vi "Read Gain Values.vi"(6 "error in":errorcluster, 8 "MaxRead":i32, 9 "Channel in":u16) -> (0 "error out":errorcluster, 1 "Messages":T2(array[cluster]) {"ID" format="%.0x"; "DATA[0]" format="%.0x"; "DATA[1]" format="%.0x"; "DATA[2]" format="%.0x"; "DATA[3]" format="%.0x"; "DATA[4]" format="%.0x"; "DATA[5]" format="%.0x"; "DATA[6]" format="%.0x"; "DATA[7]" format="%.0x"}, 2 "Pass":bool, 3 "Channel out":u16)   [LabVIEW 2023]
uses:
  4f930f32-d09a-43ef-bca1-8b214b378bd5.vi
  e8470de1-fa2d-4ee3-b50e-96bd89dc731f.vi
  Communication/PCAN2023/PCAN API.lvlib
panel:
  out "MessageBuffer out 4":T1 {"ID" format="%.0x"; "DATA[0]" format="%.0x"; "DATA[1]" format="%.0x"; "DATA[2]" format="%.0x"; "DATA[3]" format="%.0x"; "DATA[4]" format="%.0x"; "DATA[5]" format="%.0x"; "DATA[6]" format="%.0x"; "DATA[7]" format="%.0x"}
  in  "stop 4":bool
  out "Numeric 4":i32
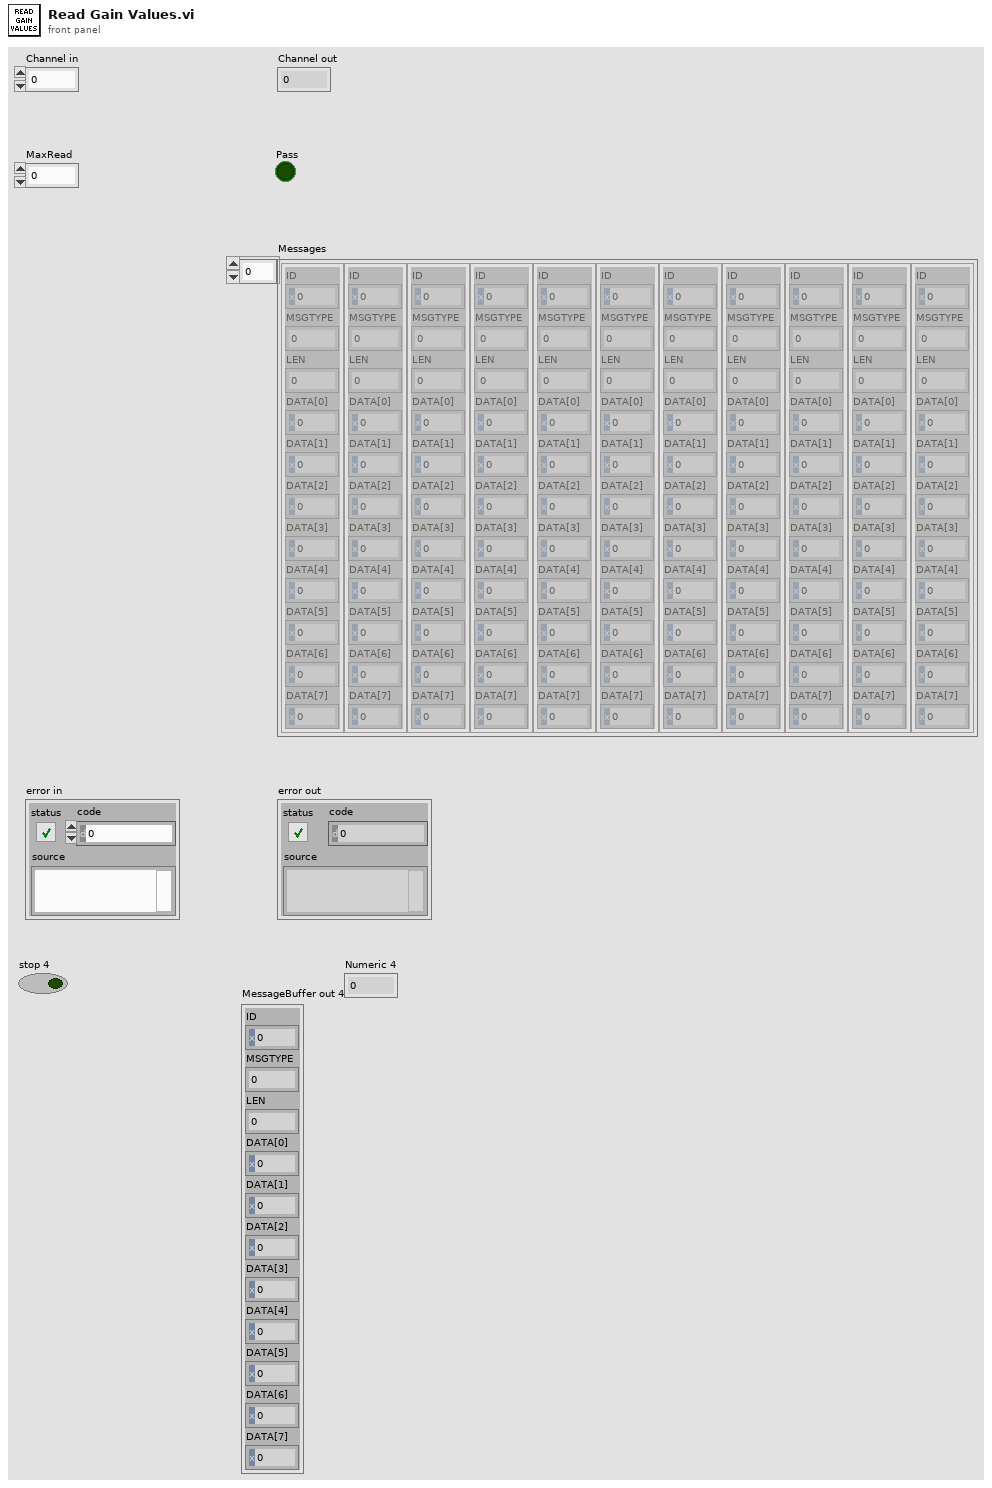
[diagram p1: front panel]
types:
  T1 = cluster{"ID":u32, "MSGTYPE":u8, "LEN":u8, "DATA[0]":u8, "DATA[1]":u8, "DATA[2]":u8, "DATA[3]":u8, "DATA[4]":u8, "DATA[5]":u8, "DATA[6]":u8, "DATA[7]":u8}
  T2 = cluster{"ID":u32, "MSGTYPE":u8, "LEN":u8, "DATA[0]":u8, "DATA[1]":u8, "DATA[2]":u8, "DATA[3]":u8, "DATA[4]":u8, "DATA[5]":u8, "DATA[6]":u8, "DATA[7]":u8}[]
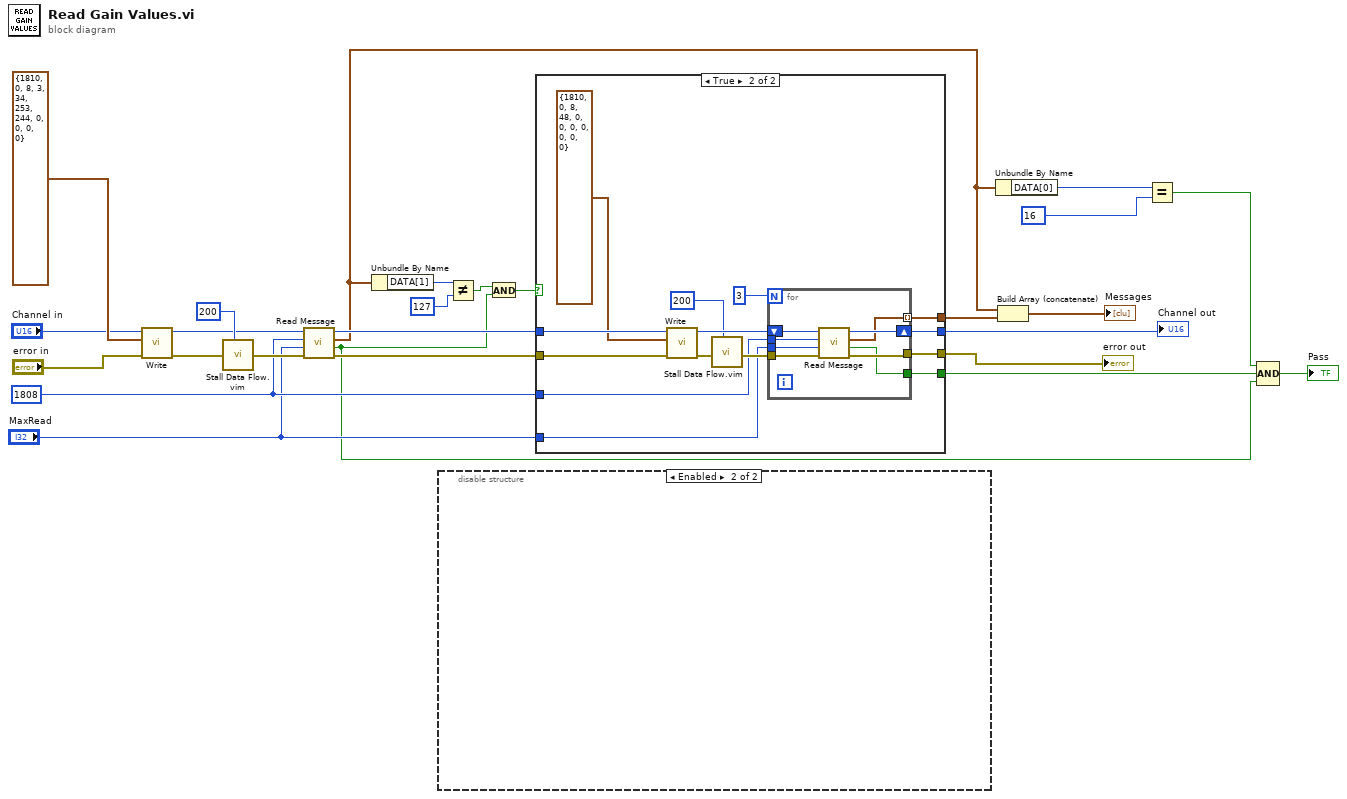
[diagram p0: block diagram]
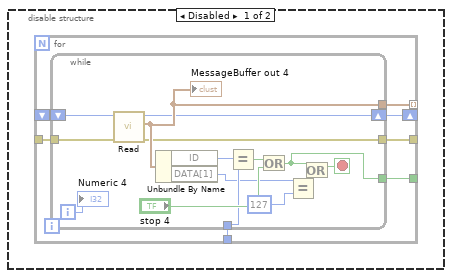
[diagram p2: hidden frame]
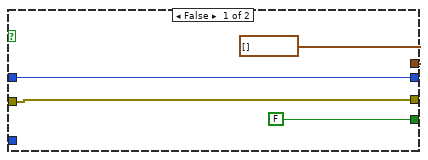
[diagram p3: hidden frame]
diagram:
  (unwired) u32 200 ("milliseconds to wait")
  w5 = u32 1808 ("ID")
  n1 = call "Write.vi"("error in"="error in", "MessageBuffer"=T1 {"ID"=1810, "MSGTYPE"=0, "LEN"=8, "DATA[0]"=3, "DATA[1]"=34, "DATA[2]"=253, "DATA[3]"=244, "DATA[4]"=0, "DATA[5]"=0, "DATA[6]"=0, "DATA[7]"=0}, "Channel"="Channel in") -> ("error out"=w21:errorcluster, "Channel out"=w10:u16)  [unwired: 5 in, 2 out]
  n2 = call "Stall Data Flow.vim"("value in"=w21, "milliseconds to wait"=u32 200) -> ("value out"=w9:errorcluster)  [unwired: 1 out]
  n3 = call "Read Message.vi"("error in"=w9, "MaxRead"="MaxRead", "ID"=w5, "Channel in"=w10) -> ("error out"=w7:errorcluster, "Passed"=w1:bool, "Last Message"=w6:T1, "Channel out"=w8:u16)  [unwired: 3 in, 1 out]
  n4 = Unbundle By Name(w6) -> ("DATA[1]"=w14:u8)
  n5 = disable-structure shown="Enabled" {
    frame Disabled {
      n6 = for {
        tunnel: _ -> [w33]
        tunnel: [w31] -> _
        shift-right: [w29] -> _
        shift-left: _ -> [w30]
        tunnel: [w27] -> _ mode=indexing
        tunnel: _ -> [w28]
        tunnel: [w32] -> _
        n7 = while {
          tunnel: w28 -> [w48]
          tunnel: w33 -> [w43]
          tunnel: [w42] -> w27
          tunnel: [w41] -> w32
          tunnel: [w34] -> w31
          shift-right: [w39] -> w29
          shift-left: w30 -> [w40]
          i -> [w44]
          stop <- w36 stop-if-true
          n8 = call "Read.vi"("error in"=w48, "Channel"=w40) -> ("error out"=w41:errorcluster, "MessageBuffer out"=w42:T1, "Channel out"=w39:u16)  [unwired: 6 in, 1 out]
          "MessageBuffer out 4" <- w42
          n9 = Unbundle By Name(w42) -> ("ID"=w47:u32, "DATA[1]"=w37:u8)
          n10 = Equal?(x=w47, y=w43) -> (x = y?=w46:bool)
          n11 = Or(x=w46, y="stop 4") -> (x .or. y?=w34:bool)
          n12 = Equal?(x=w37, y=u8 127) -> (x = y?=w35:bool)
          n13 = Or(x=w34, y=w35) -> (x .or. y?=w36:bool)
          "Numeric 4" <- w44
        }
      }
    }
    frame Enabled {
    }
  }
  n14 = Not Equal?(x=w14, y=u8 127) -> (x != y?=w3:bool)
  n15 = And(x=w3, y=w1) -> (x .and. y?=w2:bool)
  n16 = case shown="True" w2 {
    tunnel: w8 -> [w51 w66]
    tunnel: w7 -> [w50 w65]
    tunnel: [w50 w64] -> w18
    tunnel: [FALSE w63] -> w17
    tunnel: [w51 w61] -> w16
    tunnel: [T2 [] w55] -> w15
    tunnel: w5 -> [_ w54]
    tunnel: "MaxRead" -> [_ w53]
    frame False {
    }
    frame True {
      n17 = call "Write.vi"("error in"=w65, "MessageBuffer"=T1 {"ID"=1810, "MSGTYPE"=0, "LEN"=8, "DATA[0]"=48, "DATA[1]"=0, "DATA[2]"=0, "DATA[3]"=0, "DATA[4]"=0, "DATA[5]"=0, "DATA[6]"=0, "DATA[7]"=0}, "Channel"=w66) -> ("error out"=w58:errorcluster, "Channel out"=w62:u16)  [unwired: 5 in, 2 out]
      n18 = call "Stall Data Flow.vim"("value in"=w58, "milliseconds to wait"=u32 200) -> ("value out"=w60:errorcluster)  [unwired: 1 out]
      n19 = for {
        N: 3 -> [_]
        tunnel: [w69] -> w63
        shift-right: [w72] -> w61
        shift-left: w62 -> [w74]
        tunnel: [w71] -> w55 mode=indexing
        tunnel: w60 -> [w73]
        tunnel: [w70] -> w64
        tunnel: w54 -> [w68]
        tunnel: w53 -> [w67]
        n20 = call "Read Message.vi"("error in"=w73, "MaxRead"=w67, "ID"=w68, "Channel in"=w74) -> ("error out"=w70:errorcluster, "Passed"=w69:bool, "Last Message"=w71:T1, "Channel out"=w72:u16)  [unwired: 3 in, 1 out]
      }
    }
  }
  "error out" <- w18
  "Channel out" <- w16
  n21 = Unbundle By Name(w6) -> ("DATA[0]"=w20:u8)
  n22 = Build Array (concatenate)(w6, w15) -> (→"Messages":T2)
  n23 = Equal?(x=w20, y=u8 16) -> (x = y?=w12:bool)
  n24 = Compound Arithmetic op=AND(w12, w17, w1) -> (→"Pass":bool)
